vi "CalculateKey.vi"(11 "Seed":u8[](array[numeric]) format="%.0x") -> (2 "Key Bytes":u8[](array[numeric]) format="%.0x", 3 "Key":i32)   [LabVIEW 2021, in "Lunar UDS CAN.lvlib"]
uses:
  Lunar UDS CAN.lvlib
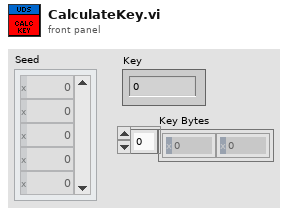
[diagram p1: front panel]
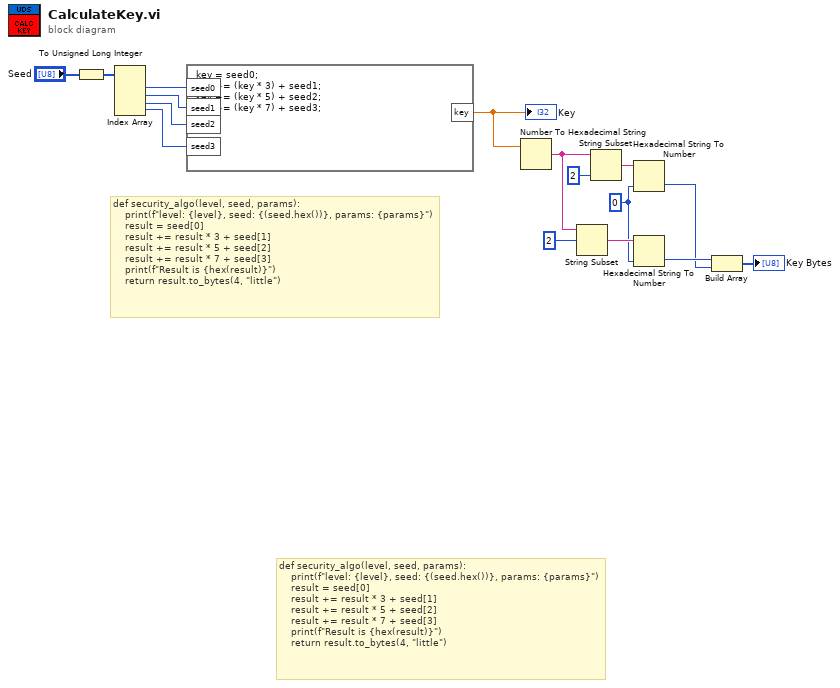
[diagram p0: block diagram]
diagram:
  w8 = u8 0 ("default (0 U32)")
  # "def security_algo(level, seed, params):\n    print(f\"level: {level}, seed: {(seed.hex())}, params: {params}\")\n    result = seed[0]\n    result += result * 3 + seed[1]\n    result += result * 5 + seed[2]\n    result += result * 7 + seed[3]\n    print(f\"Result is {hex(result)}\")\n    return result.to_bytes(4, \"little\")"
  # "def security_algo(level, seed, params):\n    print(f\"level: {level}, seed: {(seed.hex())}, params: {params}\")\n    result = seed[0]\n    result += result * 3 + seed[1]\n    result += result * 5 + seed[2]\n    result += result * 7 + seed[3]\n    print(f\"Result is {hex(result)}\")\n    return result.to_bytes(4, \"little\")"
  n1 = To Unsigned Long Integer(number="Seed") -> (unsigned 32bit integer=w15:u32[])
  n2 = Index Array(array=w15) -> (element #1=w7:u32, element #2=w6:u32, element #3=w5:u32, element #4=w4:u32)  [unwired: 4 in]
  n3 = formula code="key = seed0;\nkey += (key * 3) + seed1;\nkey += (key * 5) + seed2;\nkey += (key * 7) + seed3;"("seed0"=w7, "seed1"=w6, "seed2"=w5, "seed3"=w4) -> ("key"=w3:dbl)
  "Key" <- w3
  n4 = Number To Hexadecimal String(2:w3) -> (0:w13:string)  [unwired: 1 in]
  n5 = String Subset(string=w13, offset (0)=2) -> (substring=w10:string)  [unwired: 1 in]
  n6 = String Subset(string=w13, length (rest)=2 ("length (rest)")) -> (substring=w11:string)  [unwired: 1 in]
  n7 = Hexadecimal String To Number(string=w11, default (0uL)=w8) -> (number=w1:u8)  [unwired: 1 in, 1 out]
  n8 = Hexadecimal String To Number(string=w10, default (0uL)=w8) -> (number=w2:u8)  [unwired: 1 in, 1 out]
  n9 = Build Array(w2, w1) -> (→"Key Bytes":u8[])
